vi "Histogram calculation and plotting.vi"() -> ()   [LabVIEW 2018]
uses:
  <vilib>/gmath/statdist.llb/Normal Random.vi
  <vilib>/Analysis/NI_AALPro.lvlib
  <vilib>/gmath/NI_Gmath.lvlib
  Tracker.lvlib
  <vilib>/ptbypt/NI_PtbyPt.lvlib
panel:
  out "XY Graph":T1(graph)
  in  "Min":dbl format="%#_13g"
  in  "Max":dbl=300.0 format="%#_13g"
  in  "N bins":i32=10
  in  "Enum":enum16{"Own", "LV Full", "LV Pt-by-Pt"}(ring)
  in  "mean":dbl(knob)=125.0 scale=0.0..300.0
  in  "std":dbl(knob)=25.0 scale=0.0..100.0
  out "1 sample proc. time, ms":dbl format="%#_6f"
  out "1 hour proc. time, ms":dbl
  out "XY Graph - Light":T1(graph)
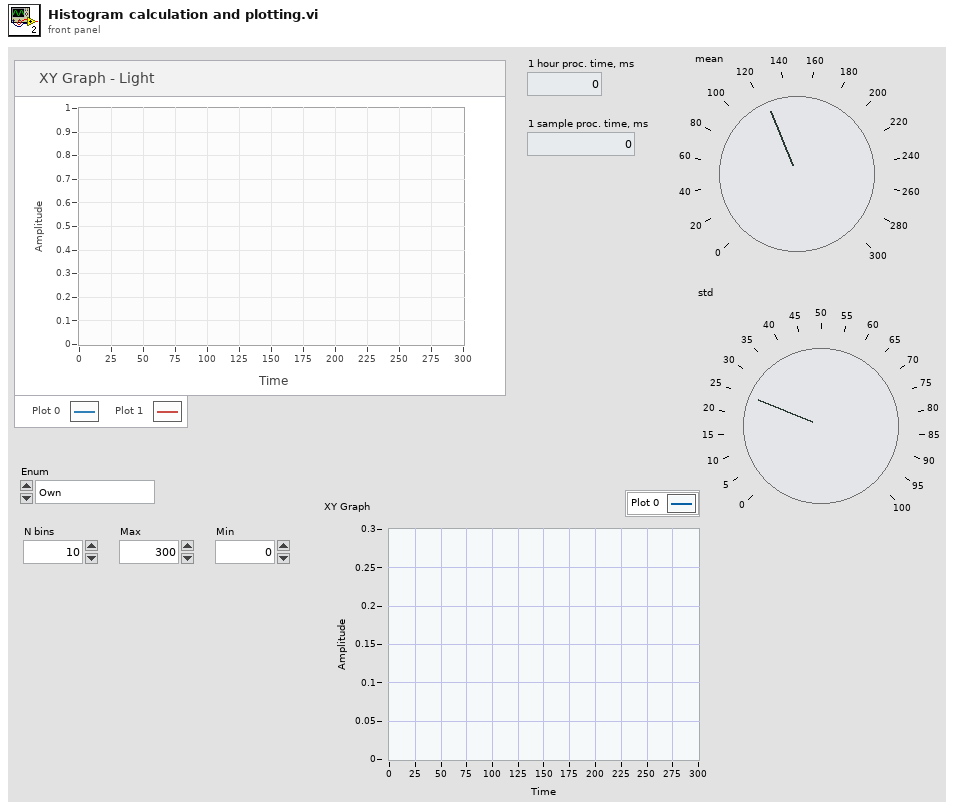
[diagram p1: front panel]
types:
  T1 = cluster{"X Values":dbl[], "Histogram: h(x)":dbl[]}
  T2 = cluster{"X Values":dbl[], "Histogram: h(x)":i32[]}
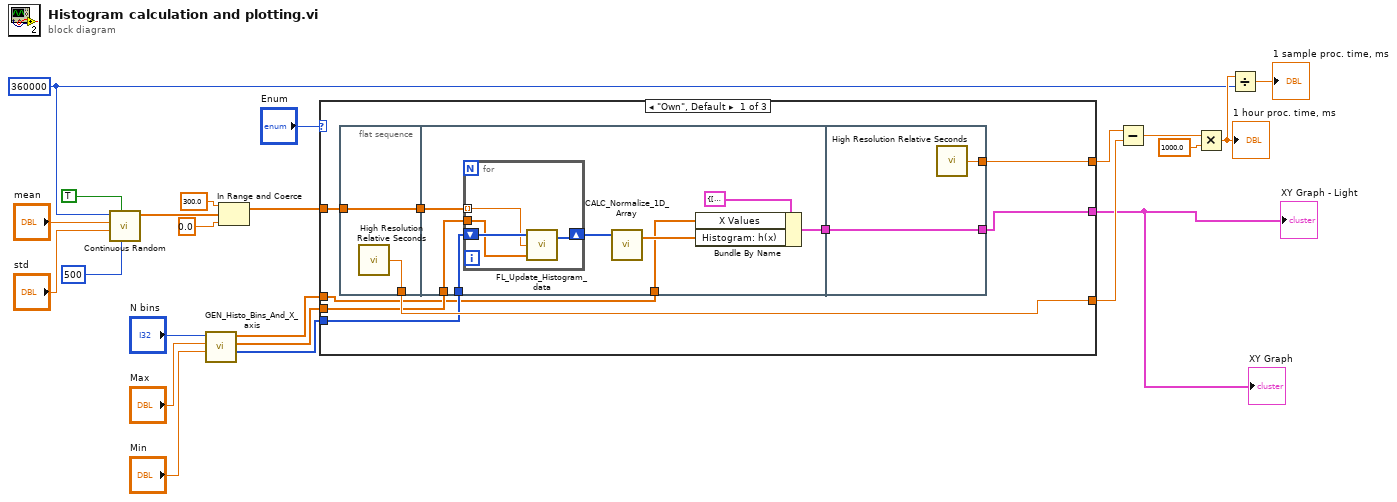
[diagram p0: block diagram]
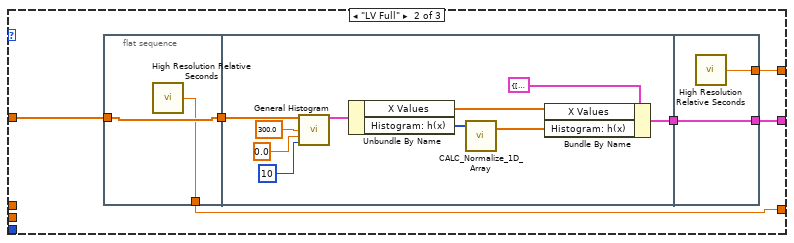
[diagram p2: hidden frame]
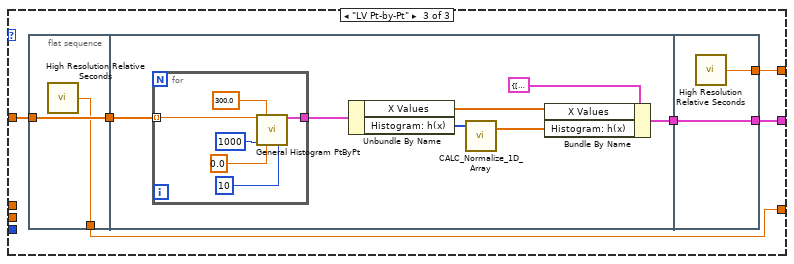
[diagram p3: hidden frame]
diagram:
  w11 = 360000 ("samples")
  n1 = call-poly <vilib>:"Continuous Random.vi"("seed"=500, "reset"=TRUE, "std"="std", "mean"="mean", "samples"=w11) -> ("normal random data"=w19:dbl[])  [unwired: 5 in, 1 out]
  n2 = call "GEN_Histo_Bins_And_X_axis.vi"("Min"="Min", "Max"="Max", "N bins"="N bins") -> ("Initial bins count"=w2:u32[], "Bins"=w3:dbl[], "X axis values"=w4:dbl[])  [unwired: 5 in, 1 out]
  n3 = In Range and Coerce(upper limit=300.0 ("min"), x=w19, lower limit=0.0 ("min")) -> (coerced(x)=w9:dbl[])  [unwired: 1 out]
  n4 = case shown="\"Own\", Default" "Enum" {
    tunnel: [w28 w52 w72] -> w16
    tunnel: [w29 w51 w71] -> w15
    tunnel: [w27 w50 w70] -> w1
    tunnel: w9 -> [w30 w49 w69]
    tunnel: w3 -> [w26 _ _]
    tunnel: w2 -> [w25 _ _]
    tunnel: w4 -> [w24 _ _]
    frame "Own", Default {
      n5 = flat-sequence {
        tunnel: [w33] -> w32
        tunnel: [w34] -> w29
        tunnel: w30 -> [w33]
        tunnel: w32 -> [w39]
        tunnel: [w40] -> w31
        tunnel: w26 -> [w38]
        tunnel: w25 -> [w37]
        tunnel: w24 -> [w35]
        tunnel: [w48] -> w28
        tunnel: [w47] -> w27
        tunnel: w31 -> [w47]
        frame #0 {
          n6 = call <vilib>:"High Resolution Relative Seconds.vi"() -> ("relative seconds"=w34:dbl)
        }
        frame #1 {
          n7 = for {
            tunnel: w39 -> [w44] mode=indexing
            tunnel: w38 -> [w45]
            shift-right: [w43] -> w36
            shift-left: w37 -> [w46]
            n8 = call "FL_Update_Histogram_data.vi"("Histogram count in"=w46, "Current value"=w44, "Bins array"=w45) -> ("Histogram count out"=w43:u32[])  [unwired: 3 in]
          }
          n9 = call "CALC_Normalize_1D_Array.vi"("1D array"=w36) -> ("Normalized 1D array"=w41:dbl[])  [unwired: 2 in, 1 out]
          n10 = Bundle By Name(cluster=T1 {"X Values"=[15.0, 45.0, 75.0, 105.0, 135.0, 165.0, 195.0, 225.0, 255.0, 285.0], "Histogram: h(x)"=[-1.0, -1.0, 0.0, 1.0, 2.0, 1.0, 0.0, -1.0, -1.0, -1.0]} ("XY Graph - Light"), "X Values"=w35, "Histogram: h(x)"=w41) -> (w40:T1)
        }
        frame #2 {
          n11 = call <vilib>:"High Resolution Relative Seconds.vi"() -> ("relative seconds"=w48:dbl)
        }
      }
    }
    frame "LV Full" {
      n12 = flat-sequence {
        tunnel: w49 -> [w56]
        tunnel: [w56] -> w54
        tunnel: [w55] -> w51
        tunnel: w54 -> [w63]
        tunnel: [w57] -> w53
        tunnel: [w68] -> w52
        tunnel: [w67] -> w50
        tunnel: w53 -> [w67]
        frame #0 {
          n13 = call <vilib>:"High Resolution Relative Seconds.vi"() -> ("relative seconds"=w55:dbl)
        }
        frame #1 {
          n14 = call <vilib>:"General Histogram.vi"("X"=w63, "max"=300.0, "min"=0.0, "# bins"=10) -> ("Histogram Graph"=w61:T2)  [unwired: 7 in, 4 out]
          n15 = Unbundle By Name(w61) -> ("X Values"=w58:dbl[], "Histogram: h(x)"=w62:i32[])
          n16 = call "CALC_Normalize_1D_Array.vi"("1D array"=w62) -> ("Normalized 1D array"=w59:dbl[])  [unwired: 2 in, 1 out]
          n17 = Bundle By Name(cluster=T1 {"X Values"=[15.0, 45.0, 75.0, 105.0, 135.0, 165.0, 195.0, 225.0, 255.0, 285.0], "Histogram: h(x)"=[-1.0, -1.0, 0.0, 1.0, 2.0, 1.0, 0.0, -1.0, -1.0, -1.0]} ("XY Graph - Light"), "X Values"=w58, "Histogram: h(x)"=w59) -> (w57:T1)
        }
        frame #2 {
          n18 = call <vilib>:"High Resolution Relative Seconds.vi"() -> ("relative seconds"=w68:dbl)
        }
      }
    }
    frame "LV Pt-by-Pt" {
      n19 = flat-sequence {
        tunnel: w69 -> [w76]
        tunnel: [w76] -> w74
        tunnel: [w75] -> w71
        tunnel: w74 -> [w78]
        tunnel: [w79] -> w73
        tunnel: [w91] -> w72
        tunnel: [w90] -> w70
        tunnel: w73 -> [w90]
        frame #0 {
          n20 = call <vilib>:"High Resolution Relative Seconds.vi"() -> ("relative seconds"=w75:dbl)
        }
        frame #1 {
          n21 = for {
            tunnel: w78 -> [w88] mode=indexing
            tunnel: [w85] -> w77
            n22 = call <vilib>:"General Histogram PtByPt.vi"("x"=w88, "max"=300.0, "sample length"=1000, "min"=0.0, "# bins"=10) -> ("Histogram Graph"=w85:T2)  [unwired: 6 in, 4 out]
          }
          n23 = Unbundle By Name(w77) -> ("X Values"=w80:dbl[], "Histogram: h(x)"=w83:i32[])
          n24 = call "CALC_Normalize_1D_Array.vi"("1D array"=w83) -> ("Normalized 1D array"=w81:dbl[])  [unwired: 2 in, 1 out]
          n25 = Bundle By Name(cluster=T1 {"X Values"=[15.0, 45.0, 75.0, 105.0, 135.0, 165.0, 195.0, 225.0, 255.0, 285.0], "Histogram: h(x)"=[-1.0, -1.0, 0.0, 1.0, 2.0, 1.0, 0.0, -1.0, -1.0, -1.0]} ("XY Graph - Light"), "X Values"=w80, "Histogram: h(x)"=w81) -> (w79:T1)
        }
        frame #2 {
          n26 = call <vilib>:"High Resolution Relative Seconds.vi"() -> ("relative seconds"=w91:dbl)
        }
      }
    }
  }
  "XY Graph - Light" <- w1
  "XY Graph" <- w1
  n27 = Subtract(x=w16, y=w15) -> (x-y=w14:dbl)
  n28 = Multiply(x=w14, y=1000.0) -> (x*y=w12:dbl)
  "1 hour proc. time, ms" <- w12
  n29 = Divide(x=w12, y=w11) -> (x/y=→"1 sample proc. time, ms":dbl)
